vi "Virtual particle trace (backward).vi"(6 "U_inf":sgl[](array[numeric])=[1.0, 0.0, 0.0], 8 "r_max":sgl=10.0, 9 "dt":sgl=0.01, 10 "P_start":sgl[](array[numeric])=[0.0, 0.0, 0.0], 11 "Panel triangles in":T1[](array[typedef])) -> (0 "W":sgl[](array[numeric]), 1 "V":sgl[](array[numeric]), 2 "U":sgl[](array[numeric]), 3 "r":sgl[](array[numeric]), 4 "Completed":bool, 5 "Points":sgl[][](array[numeric]))   [LabVIEW 2017]
uses:
  ctls/Triangle panel.ctl
panel:
  out "r / r_max":sgl
  out "Progress":sgl(slide)=3330.0 scale=0.0..3330.0
  out "loop number":i32
  in  "Stop":bool
  # "If progress bar stops advancing while loop number continues increasing, press stop to exit the loop."
  # "Lack of progress is caused by a particle getting \"stuck\"."
  # "PN 26/10/17"
  # "Vertices"
  # "Edges"
  # "Unit normal"
  # "Control point"
  # "Edge\nlinks \n(tri index)"
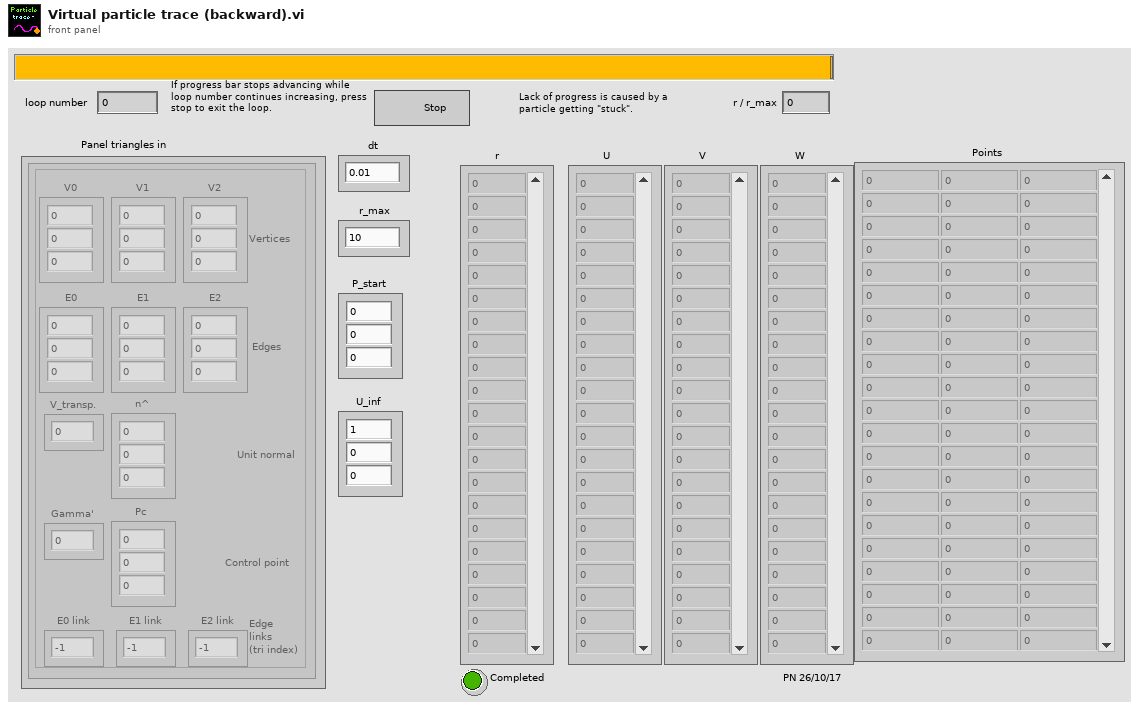
[diagram p1: front panel]
types:
  T1 = typedef "Triangle panel.ctl" = cluster{"V0":sgl[], "V1":sgl[], "V2":sgl[], "E0":sgl[], "E1":sgl[], "E2":sgl[], "n^":sgl[], "Pc":sgl[], "Gamma'":sgl, "V_transp.":sgl, "E0 link":i32, "E1 link":i32, "E2 link":i32}
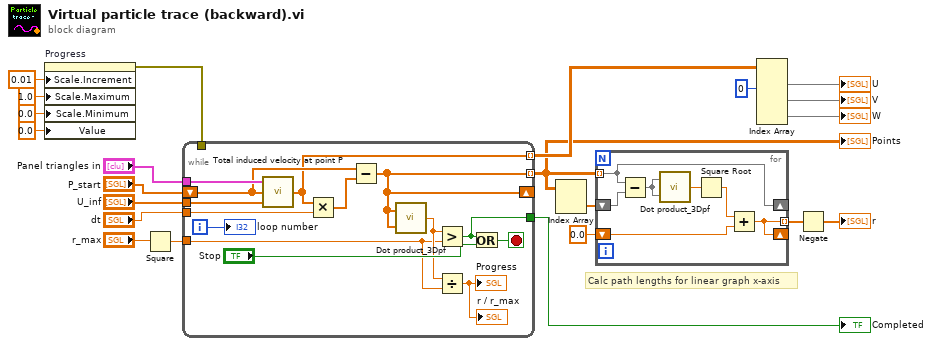
[diagram p0: block diagram]
diagram:
  # "Calc path lengths for linear graph x-axis"
  n1 = property on="Progress" class="Slide (strict)"("Scale.Increment"=0.01 ("Scale.Range:Increment"), "Scale.Maximum"=1.0 ("Scale.Range:Maximum"), "Scale.Minimum"=0.0 ("Scale.Range:Minimum"), "Value"=sgl 0.0 ("Progress")) -> (error out=w8:errorcluster)  [unwired: 2 in, 1 out]
  n2 = Square(x="r_max") -> (x^2=w13:sgl)
  n3 = while {
    tunnel: "U_inf" -> [w36]
    tunnel: "Panel triangles in" -> [w35]
    shift-right: [w27] -> _
    shift-left: "P_start" -> [w34]
    tunnel: "dt" -> [w33]
    tunnel: [w27] -> w1 mode=indexing
    tunnel: w13 -> [w25]
    tunnel: [w30] -> w17 mode=indexing
    tunnel: w8 -> [_]
    tunnel: [w23] -> w3
    i -> [w31]
    stop <- w29 stop-if-true
    n4 = call "Total induced velocity at point P.vi"("U_inf"=w36, "P"=w34, "Triangle panels"=w35) -> ("(U, V, W) at P"=w30:sgl[])
    n5 = Multiply(x=w30, y=w33) -> (x*y=w32:sgl[])
    n6 = Subtract(x=w34, y=w32) -> (x-y=w27:sgl[])
    n7 = call "Dot product_3Dpf.vi"("B"=w27, "A"=w27) -> ("A . B"=w26:sgl)
    n8 = Greater?(x=w26, y=w25) -> (0:w23:bool)
    n9 = Divide(x=w26, y=w25) -> (x/y=→"Progress" →"r / r_max":sgl)
    n10 = Or(x=w23, y="Stop") -> (x .or. y?=w29:bool)
    "loop number" <- w31
  }
  "Completed" <- w3
  "Points" <- w1
  n11 = Index Array(array=w1) -> (element=w19:sgl[])  [unwired: 2 in]
  n12 = for {
    tunnel: w1 -> [w39] mode=indexing
    shift-right: [w39] -> _
    shift-left: w19 -> [w43]
    tunnel: [w37] -> w4 mode=indexing
    shift-right: [w37] -> _
    shift-left: sgl 0.0 -> [w38]
    n13 = Subtract(x=w39, y=w43) -> (x-y=w42:sgl[])
    n14 = call "Dot product_3Dpf.vi"("B"=w42, "A"=w42) -> ("A . B"=w41:sgl)
    n15 = Square Root(x=w41) -> (sqrt(x)=w40:sgl)
    n16 = Add(x=w40, y=w38) -> (x+y=w37:sgl)
  }
  n17 = Index Array(array=w17, index (col) #1=0 ("disabled index (col)")) -> (element #1=→"U":sgl[], element #2=→"V":sgl[], element #3=→"W":sgl[])  [unwired: 5 in]
  n18 = Negate(x=w4) -> (-x=→"r":sgl[])
